vi "I-O Test_Kai.vi"() -> ()   [LabVIEW 2021, in "Test VIs.lvclass"]
uses:
  Test VIs/Test VIs.lvclass
  Classes/Controller/I-O/I-O.lvclass
  Classes/Controller/Controller.lvclass
panel:
  out "Compression Sensor":bool=TRUE
  out "Sensor Channel":dbl
  out "Sensor":bool=TRUE
  out "sensor pin number":i32
  out "tray sensor":bool
  out "secondary valve sensor":bool
  out "primary valve sensor":bool
  in  "Turn on secondary vacuum":bool
  in  "turn on primary vacuum":bool
  in  "secure tray":bool
  out "Valve Channel":dbl
  in  "Type":enum16{"O ring Vac", "Baseplate Vac"}(ring)
  in  "Position":i32
  in  "Region":i32
  in  "On/Off":bool
  in  "Stop":bool
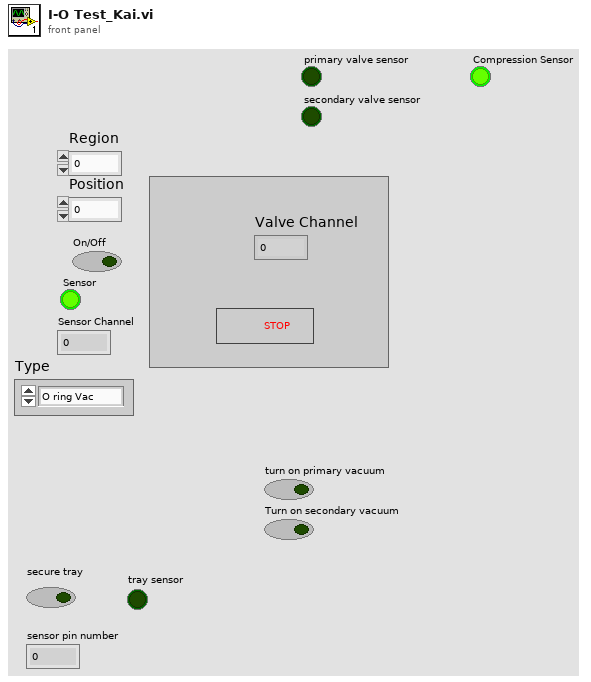
[diagram p1: front panel]
types:
  T1 = typedef "Controller.lvclass/Controllers.ctl" = cluster{"I-O.lvclass":refnum<class "I-O.lvclass">, "Gantry":refnum<k24>, "Dispenser":refnum<visa-resource-name>}
  T2 = typedef "I-O.lvclass/Pin Map.ctl" = cluster{"Region Valves":i32[], "Extra Valves":dbl[][][], "Tool Primary Valve":i32, "Tool Secondary Valve":i32, "Region Sensors":i32[], "Extra Sensors":dbl[][][], "Tool Primary Sensor":dbl, "Tool Secondary Sensor":dbl, "Compression Sensor":dbl, "5V":i32, "Dispenser Sensor":dbl, "Light Curtain":i32}
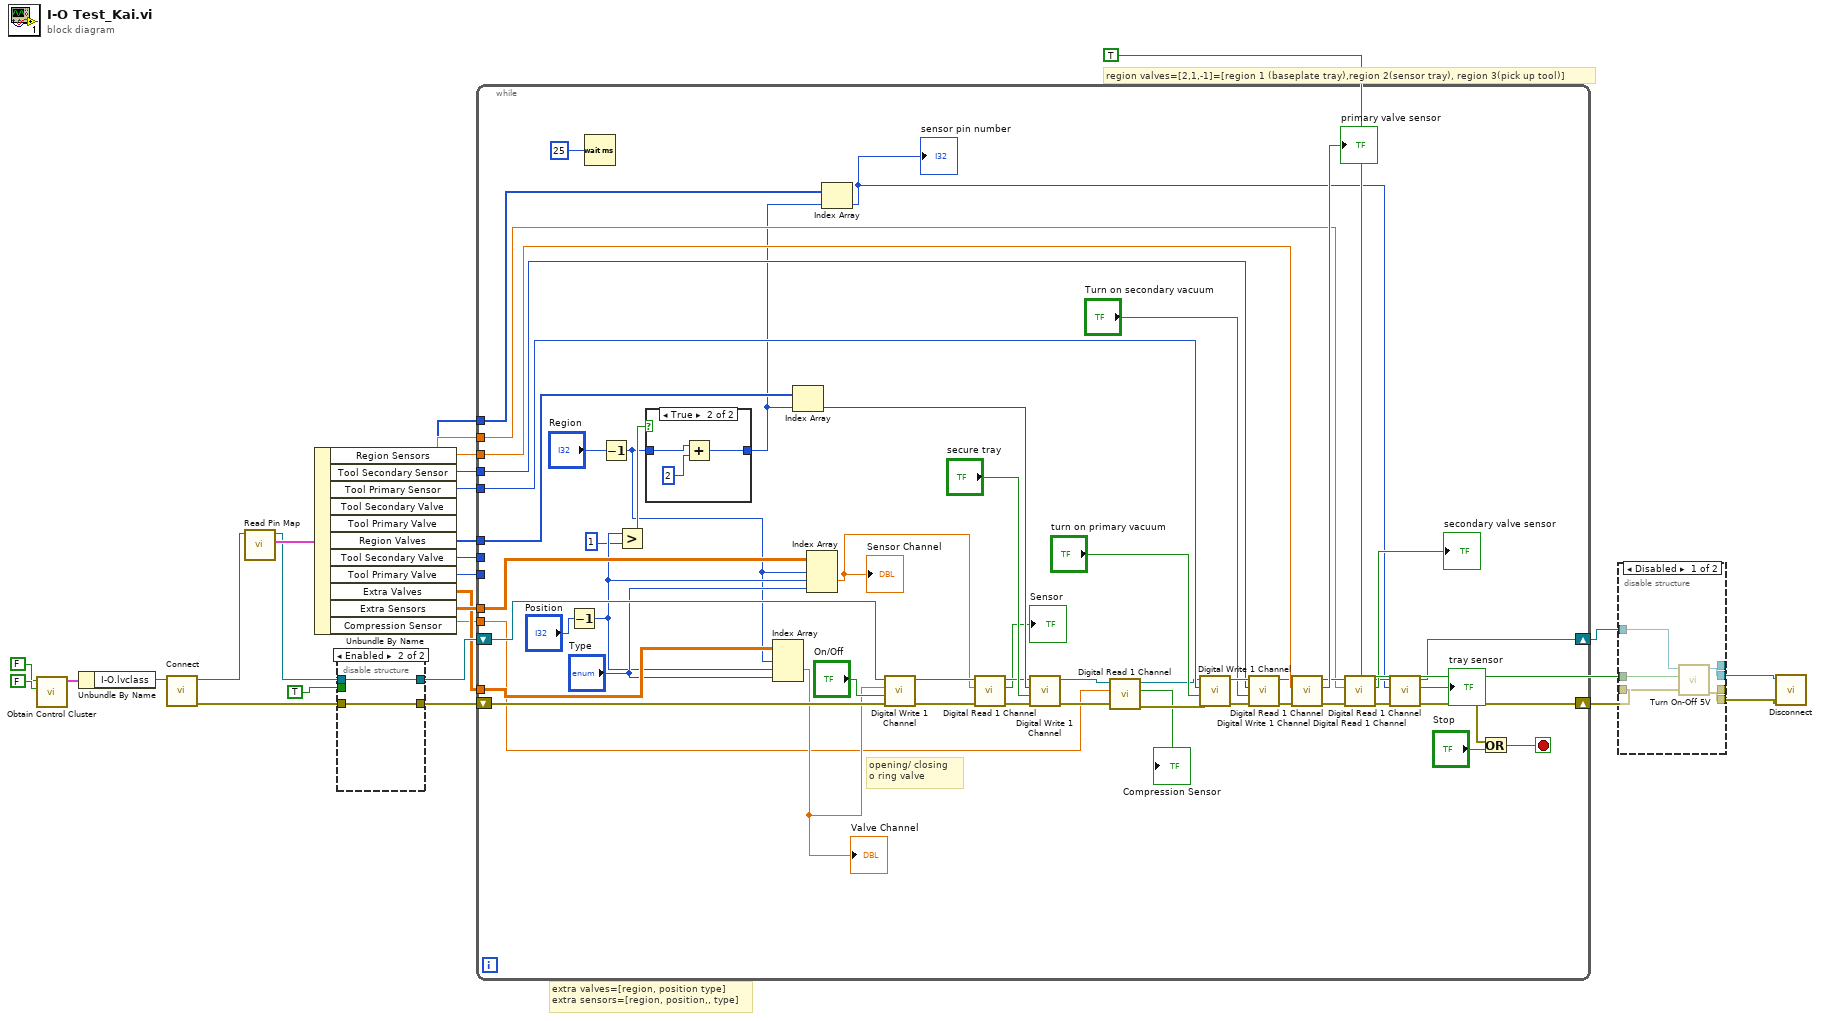
[diagram p0: block diagram]
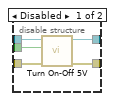
[diagram p2: hidden frame]
diagram:
  # "extra valves=[region, position type]\nextra sensors=[region, position,, type]"
  # "region valves=[2,1,-1]=[region 1 (baseplate tray),region 2(sensor tray), region 3(pick up tool)]"
  n1 = call "Obtain Control Cluster.vi"("Dispense"=FALSE, "Motion"=FALSE) -> ("Control Out"=w15:T1)  [unwired: 8 in, 1 out]
  n2 = Unbundle By Name(w15) -> ("I-O.lvclass"=w14:refnum<class "I-O.lvclass">)
  n3 = call-dynamic "Connect.vi"("Controller in"=w14) -> ("error out"=w20:errorcluster, "Controller out"=w22:refnum<class "I-O.lvclass">)  [unwired: 9 in]
  n4 = call-dynamic "Read Pin Map.vi"("I-O in"=w22) -> ("Pin Map 2"=w24:T2, "I-O out"=w23:refnum<class "I-O.lvclass">)  [unwired: 8 in, 1 out]
  n5 = Unbundle By Name(w24) -> ("Region Sensors"=w5:i32[], "Tool Secondary Sensor"=w6:dbl, "Tool Primary Sensor"=w7:dbl, "Tool Secondary Valve"=w8:i32, "Tool Primary Valve"=w9:i32, "Region Valves"=w10:i32[], "Tool Secondary Valve"=w12:i32, "Tool Primary Valve"=w11:i32, "Extra Valves"=w18:dbl[][][], "Extra Sensors"=w21:dbl[][][], "Compression Sensor"=w13:dbl)
  n6 = disable-structure shown="Enabled" {
    disable-tunnel: [w32 w34] -> w27
    disable-tunnel: TRUE ("Value") -> [w31 _]
    disable-tunnel: w23 -> [w30 w34]
    disable-tunnel: w20 -> [w29 w33]
    disable-tunnel: [w28 w33] -> w19
    frame Disabled {
      n7 = call-dynamic "Turn On-Off 5V.vi"("error in (no error)"=w29, "Value"=w31, "I-O in"=w30) -> ("error out"=w28:errorcluster, "I-O out"=w32:refnum<class "I-O.lvclass">)  [unwired: 7 in]
    }
    frame Enabled {
    }
  }
  n8 = while {
    shift-right: [w57] -> w25
    shift-left: w27 -> [w84]
    tunnel: w21 -> [w48]
    shift-right: [w59] -> w4
    shift-left: w19 -> [w83]
    tunnel: w18 -> [w49]
    tunnel: w13 -> [w41]
    tunnel: w12 -> [_]
    tunnel: w11 -> [_]
    tunnel: w10 -> [w78]
    tunnel: w9 -> [w75]
    tunnel: w8 -> [w72]
    tunnel: w7 -> [w69]
    tunnel: w6 -> [w64]
    tunnel: w5 -> [w61]
    stop <- w85 stop-if-true
    # "opening/ closing \no ring valve"
    n9 = Decrement(x="Position") -> (x-1=w39:i32)
    n10 = Wait (ms)(milliseconds to wait=u32 25) -> ()  [unwired: 1 out]
    n11 = Decrement(x="Region") -> (x-1=w36:i32)
    n12 = Greater?(x=w39, y=1) -> (0:w37:bool)
    n13 = case shown="True" w37 {
      tunnel: w36 -> [w88 w91]
      tunnel: [w88 w90] -> w35
      frame False {
      }
      frame True {
        n14 = Add(x=w91, y=2) -> (x+y=w90:i32)
      }
    }
    n15 = Index Array "Index Array"(array=w49, index (dim 0)=w36, index (dim 1)=w39, index (dim 2)="Type") -> (element=w79:dbl)
    "Valve Channel" <- w79
    n16 = Index Array(array=w78, index=w35) -> (element=w77:i32)
    n17 = Index Array(array=w48, index (dim 0)=w36, index (dim 1)=w39, index (dim 2)="Type") -> (element=w46:dbl)
    "Sensor Channel" <- w46
    n18 = Index Array(array=w61, index=w35) -> (element=w56:i32)
    "sensor pin number" <- w56
    n19 = call-dynamic "Digital Write 1 Channel.vi"("error constant"=w83, "Value"="On/Off", "Channel"=w79, "I-O.lvclass"=w84) -> ("error IO"=w53:errorcluster, "I-O.lvclass 2"=w54:refnum<class "I-O.lvclass">)  [unwired: 6 in]
    n20 = call-dynamic "Digital Read 1 Channel.vi"("error in (no error)"=w53, "Read"=w46, "I-O in"=w54) -> ("error out"=w52:errorcluster, "Value"=→"Sensor":bool, "I-O out"=w51:refnum<class "I-O.lvclass">)  [unwired: 6 in]
    n21 = call-dynamic "Digital Write 1 Channel.vi"("error constant"=w52, "Value"="secure tray", "Channel"=w77, "I-O.lvclass"=w51) -> ("error IO"=w45:errorcluster, "I-O.lvclass 2"=w44:refnum<class "I-O.lvclass">)  [unwired: 6 in]
    n22 = call-dynamic "Digital Read 1 Channel.vi"("error in (no error)"=w45, "Read"=w41, "I-O in"=w44) -> ("error out"=w42:errorcluster, "Value"=→"Compression Sensor":bool, "I-O out"=w43:refnum<class "I-O.lvclass">)  [unwired: 6 in]
    n23 = call-dynamic "Digital Write 1 Channel.vi"("error constant"=w42, "Value"="turn on primary vacuum", "Channel"=w75, "I-O.lvclass"=w43) -> ("error IO"=w70:errorcluster, "I-O.lvclass 2"=w73:refnum<class "I-O.lvclass">)  [unwired: 6 in]
    n24 = call-dynamic "Digital Write 1 Channel.vi"("error constant"=w70, "Value"="Turn on secondary vacuum", "Channel"=w72, "I-O.lvclass"=w73) -> ("error IO"=w66:errorcluster, "I-O.lvclass 2"=w68:refnum<class "I-O.lvclass">)  [unwired: 6 in]
    n25 = call-dynamic "Digital Read 1 Channel.vi"("error in (no error)"=w66, "Read"=w69, "I-O in"=w68) -> ("error out"=w62:errorcluster, "Value"=→"primary valve sensor":bool, "I-O out"=w65:refnum<class "I-O.lvclass">)  [unwired: 6 in]
    n26 = call-dynamic "Digital Read 1 Channel.vi"("error in (no error)"=w62, "Read"=w64, "I-O in"=w65) -> ("error out"=w60:errorcluster, "Value"=→"secondary valve sensor":bool, "I-O out"=w58:refnum<class "I-O.lvclass">)  [unwired: 6 in]
    n27 = call-dynamic "Digital Read 1 Channel.vi"("error in (no error)"=w60, "Read"=w56, "I-O in"=w58) -> ("error out"=w59:errorcluster, "Value"=→"tray sensor":bool, "I-O out"=w57:refnum<class "I-O.lvclass">)  [unwired: 6 in]
    n28 = Or(x=w59, y="Stop") -> (x .or. y?=w85:bool)
  }
  n29 = disable-structure shown="Disabled" {
    disable-tunnel: [_ w98] -> _
    disable-tunnel: w25 -> [w94 w98]
    disable-tunnel: [_ w97] -> _
    disable-tunnel: w4 -> [w96 w97]
    disable-tunnel: TRUE ("Value") -> [w95 _]
    disable-tunnel: [w93 _] -> w2
    disable-tunnel: [w92 _] -> w1
    frame Disabled {
      n30 = call-dynamic "Turn On-Off 5V.vi"("error in (no error)"=w96, "Value"=w95, "I-O in"=w94) -> ("error out"=w93:errorcluster, "I-O out"=w92:refnum<class "I-O.lvclass">)  [unwired: 7 in]
    }
    frame Enabled {
    }
  }
  n31 = call-dynamic "Disconnect.vi"("error in (no error)"=w2, "I-O in"=w1) -> ()  [unwired: 8 in, 1 out]
